vi "SetTrigger.vi"(8 "error in (no error)":errorcluster, 9 "Level":dbl format="%#_13g", 10 "trigger source (External)":i32(ring)=1 items=["External"=1, "Immediate"=2, "Software"=3, "AC Line"=4, "Video"=5], 11 "KeysightN9020B in":refnum<class "KeysightN9020B.lvclass">) -> (0 "error out":errorcluster, 3 "KeysightN9020B out":refnum<class "KeysightN9020B.lvclass">)   [LabVIEW 2023, in "KeysightN9020B.lvlib" / "KeysightN9020B.lvclass"]
uses:
  KeysightN9020B.lvclass
  C:/Program Files/National Instruments/LabVIEW 2023/vi.lib/ActorFramework/Actor/Actor.lvclass
  <vilib>/ActorFramework/Actor/Actor.lvclass/Actor.ctl
  KeysightN9020B.lvclass/KeysightN9020B.ctl
  <vilib>/ActorFramework/Message Enqueuer/Message Enqueuer.lvclass/Message Enqueuer.ctl
  <vilib>/ActorFramework/Message Enqueuer/Enqueue.vi
  Interfaces/AbstractInstrumentClasses/SpectrumAnalyzer_LV/SpectrumAnalyzerComm Messages/TriggerSet Msg/TriggerSet Msg.lvclass
  C:/Program Files/National Instruments/LabVIEW 2023/vi.lib/ActorFramework/Message/Message.lvclass
  <vilib>/ActorFramework/Message Priority Queue/Priority Enqueue.vi
  <instrlib>/Keysight XSAn/Keysight XSAn.lvlib
  <vilib>/ActorFramework/Actor/Actor.lvclass
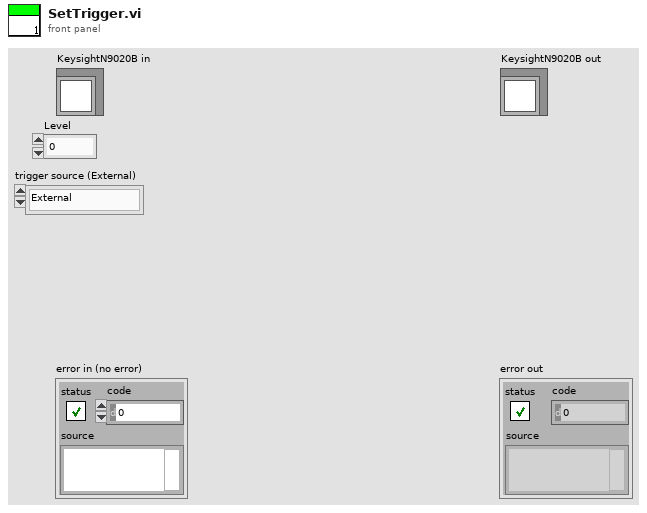
[diagram p1: front panel]
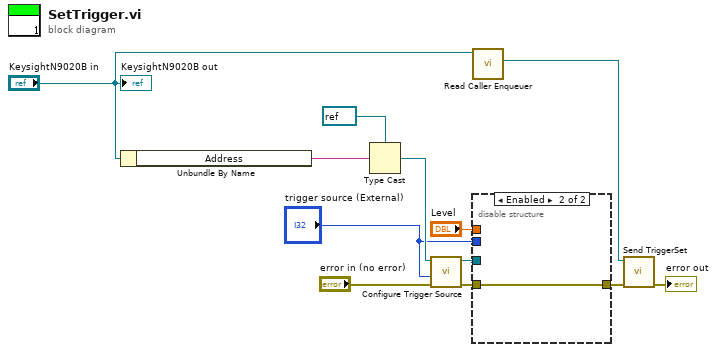
[diagram p0: block diagram]
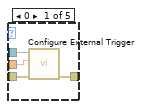
[diagram p3: hidden frame]
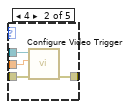
[diagram p4: hidden frame]
diagram:
  n1 = Unbundle By Name("KeysightN9020B in") -> ("Address"=w12:string)
  n2 = Type Cast(type=refnum<k15> refnum ("instrument handle"), x=w12) -> (*(type *) &x=w10:refnum<k15>)
  n3 = call <instrlib>:"Configure Trigger Source.vi"("error in (no error)"="error in (no error)", "trigger source (External)"="trigger source (External)", "instrument handle"=w10) -> ("error out"=w6:errorcluster, "instrument handle out"=w7:refnum<k15>)  [unwired: 7 in]
  n4 = call <vilib>:"Read Caller Enqueuer.vi"("Actor"="KeysightN9020B in") -> ("Caller Enqueuer"=w5:refnum<class "Message Enqueuer.lvclass">)  [unwired: 10 in]
  n5 = disable-structure shown="Enabled" {
    disable-tunnel: "Level" -> [w17 _]
    disable-tunnel: w7 -> [w16 _]
    disable-tunnel: w6 -> [w15 w29]
    disable-tunnel: [w14 w29] -> w4
    disable-tunnel: "trigger source (External)" -> [w13 _]
    frame Disabled {
      n6 = case shown="1" w13 {
        tunnel: w17 -> [w21 w25 _ _ _]
        tunnel: w16 -> [w20 w24 _ _ _]
        tunnel: w15 -> [w18 w23 w26 w27 w28]
        tunnel: [w19 w22 w26 w27 w28] -> w14
        frame 0 {
          n7 = call <instrlib>:"Configure External Trigger.vi"("error in (no error)"=w18, "external trigger level"=w21, "instrument handle"=w20) -> ("error out"=w19:errorcluster)  [unwired: 7 in, 1 out]
        }
        frame 4 {
          n8 = call <instrlib>:"Configure Video Trigger.vi"("error in (no error)"=w23, "video trigger level"=w25, "instrument handle"=w24) -> ("error out"=w22:errorcluster)  [unwired: 7 in, 1 out]
        }
        frame 1 {
        }
        frame 2 {
        }
        frame 3 {
        }
      }
    }
    frame Enabled {
    }
  }
  n9 = call "Send TriggerSet.vi"("error in (no error)"=w4, "Message Enqueuer"=w5) -> ("error out"=→"error out":errorcluster)  [unwired: 8 in, 1 out]
  "KeysightN9020B out" <- "KeysightN9020B in"
